vi "String_to_U16.vi"(6 "error in (no error)":errorcluster, 9 "String":string) -> (0 "error out":errorcluster, 3 "rest of the binary string":string, 4 "number":u16)   [LabVIEW 2015, in "Ion Motion Roboclaw.lvlib"]
uses:
  <instrlib>/Ion Motion Roboclaw/Ion Motion Roboclaw.lvlib
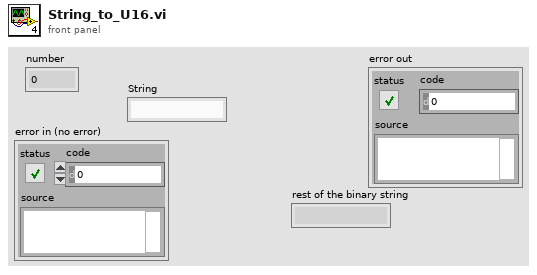
[diagram p1: front panel]
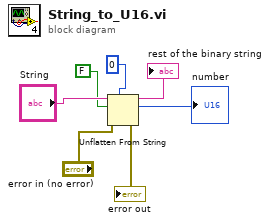
[diagram p0: block diagram]
diagram:
  n1 = Unflatten From String(type=u16 0, binary string="String", data includes array or string size? (T)=FALSE, error in (no error)="error in (no error)") -> (rest of the binary string=→"rest of the binary string":string, value=→"number":u16, error out=→"error out":errorcluster)  [unwired: 1 in]
